vi "数据输出.vi"(8 "error in (no error)":errorcluster caption="错误输入（无错误）", 11 "SingleStepTestV3 输入":refnum<class "SingleStepTestV3.lvclass">) -> (0 "error out":errorcluster caption="错误输出", 2 "数组":u16[](array[numeric]), 3 "SingleStepTestV3 输出":refnum<class "SingleStepTestV3.lvclass">)   [LabVIEW 2016, in "SingleStepTestV3.lvlib" / "SingleStepTestV3.lvclass"]
uses:
  SingleStepTestV3.lvclass
  SingleStepTestV3.lvclass/SingleStepTestV3.ctl
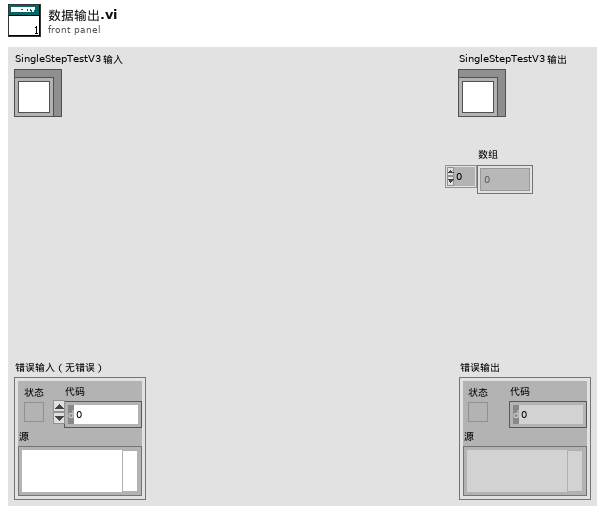
[diagram p1: front panel]
types:
  T1 = typedef "SingleStepTestV3.lvlib/SingleStepTestV3.lvclass/State Data.ctl" = cluster{"data":u16[], "仪器版本":T2}
  T2 = typedef "SingleStepTestV3.lvlib/SingleStepTestV3.lvclass/仪器版本.ctl" = enum16{"A版", "B版", "A1版"}
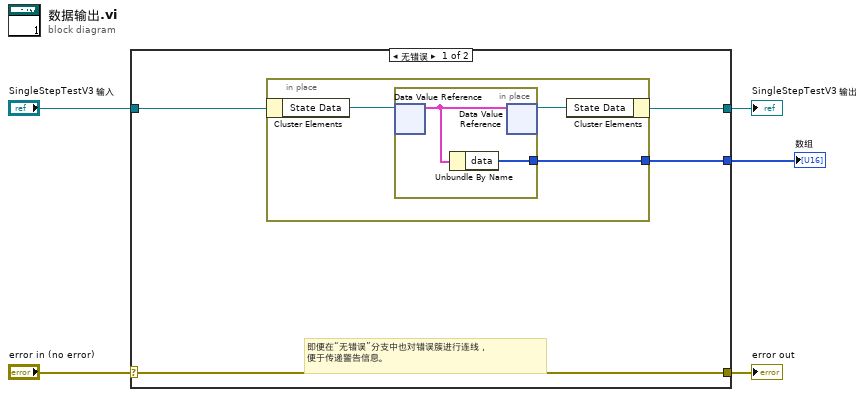
[diagram p0: block diagram]
diagram:
  n1 = case shown="无错误" "error in (no error)" {
    selector: "error in (no error)" -> [w9 w16]
    tunnel: [w9 w16] -> w4
    tunnel: [w7 w15] -> w2
    tunnel: "SingleStepTestV3 输入" -> [w8 w15]
    tunnel: [w6 _] -> w1
    frame No Error {
      # "即便在“无错误”分支中也对错误簇进行连线，\n便于传递警告信息。"
      n2 = in-place {
        in-place-border: [w10] -> w6
        n3 = in-place-cluster #1(w8) -> ("State Data"=w12:refnum<data-value>)
        n4 = in-place {
          in-place-border: [w13] -> w10
          n5 = in-place-dvr #2(w12) -> (w14:T1)  [unwired: 1 out]
          n6 = Unbundle By Name(w14) -> ("data"=w13:u16[])
          n7 = in-place-dvr #2(w14) -> (w11:refnum<data-value>)  [unwired: 1 out]
        }
        n8 = in-place-cluster #1("State Data"=w11) -> (w7:refnum<class "SingleStepTestV3.lvclass">)
      }
    }
    frame Error {
    }
  }
  "error out" <- w4
  "SingleStepTestV3 输出" <- w2
  "数组" <- w1
